vi "Read Sample Rate.vi"(0 "VISA resource name":refnum<visa-resource-name>, 11 "error in (no error)":errorcluster) -> (4 "VISA resource name out":refnum<visa-resource-name>, 6 "Delta T":dbl format="%.2e", 15 "error out":errorcluster)   [LabVIEW 2013, in "Yokogawa PZ4000.lvlib"]
doc: "This VI reads the Sample Rate of waveform for the PZ4000 series."
uses:
  <instrlib>/Yokogawa PZ4000/Yokogawa PZ4000.lvlib
panel:
  # "s"
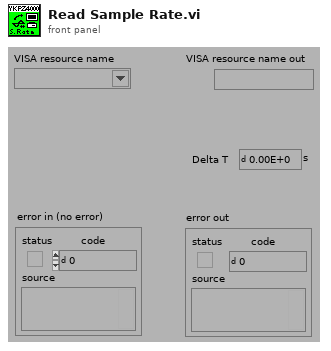
[diagram p1: front panel]
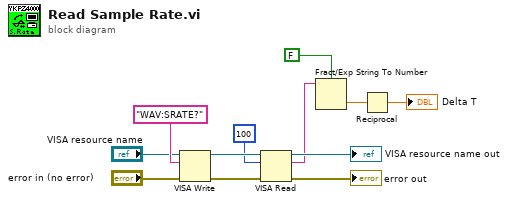
[diagram p0: block diagram]
diagram:
  n1 = VISA Write(VISA resource name="VISA resource name", write buffer="WAV:SRATE?", error in (no error)="error in (no error)") -> (VISA resource name out=w7:refnum<visa-resource-name>, error out=w11:errorcluster)  [unwired: 1 out]
  n2 = VISA Read(VISA resource name=w7, byte count=100, error in (no error)=w11) -> (VISA resource name out=→"VISA resource name out":refnum<visa-resource-name>, read buffer=w2:string, error out=→"error out":errorcluster)  [unwired: 1 out]
  n3 = Fract/Exp String To Number(use system decimal point (T)=FALSE ("¼½ÃÑ10i¬_ðgp(T)"), string=w2) -> (number=w4:dbl)  [unwired: 2 in, 1 out]
  n4 = Reciprocal(x=w4) -> (1/x=→"Delta T":dbl)
